vi "webcam to PID.vi"() -> ()   [LabVIEW 2018]
panel:
  out "output":dbl
  in  "stop":bool
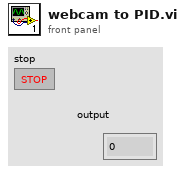
[diagram p1: front panel]
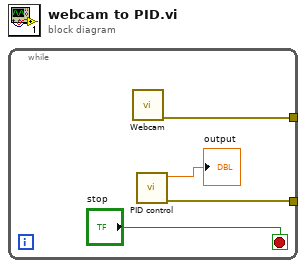
[diagram p0: block diagram]
diagram:
  n1 = while {
    tunnel: [w4] -> _
    tunnel: [w3] -> _
    stop <- "stop" stop-if-true
    n2 = call "Webcam.vi"() -> ("error out"=w3:errorcluster)  [unwired: 9 in, 1 out]
    n3 = call "PID control.vi"() -> ("error out"=w4:errorcluster, "output"=→"output":dbl)  [unwired: 10 in]
  }
